vi "Read All.vi"(8 "error in (no error)":errorcluster, 11 "Flip Mirror Containter in":refnum<class "Flip Mirror Containter.lvclass">) -> (0 "error out":errorcluster, 2 "Mirrors-NP":T1, 3 "Flip Mirror Containter out":refnum<class "Flip Mirror Containter.lvclass">)   [LabVIEW 2016, in "Flip Mirror Containter.lvclass"]
uses:
  Flip Mirror Containter.lvclass
  Controls/Flip Mirrors.ctl
  Controls/Mirror Data.ctl
  Flip Mirror Containter.lvclass/Flip Mirror Containter.ctl
  SolarMir.lvclass
  ExtFlatMir.lvclass
  ThArMir.lvclass
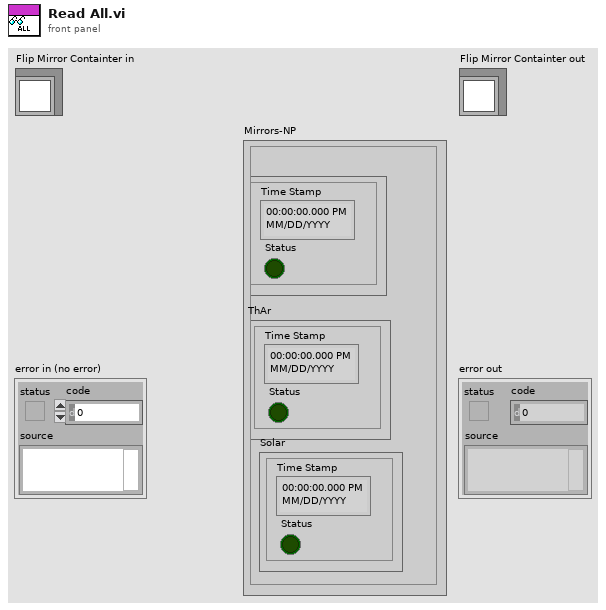
[diagram p1: front panel]
types:
  T1 = typedef "Flip Mirrors.ctl" = cluster{"ExtFlat":T2, "ThAr":T2, "Solar":T2}
  T2 = typedef "Mirror Data.ctl" = cluster{"Status":bool, "Time Stamp":timestamp}
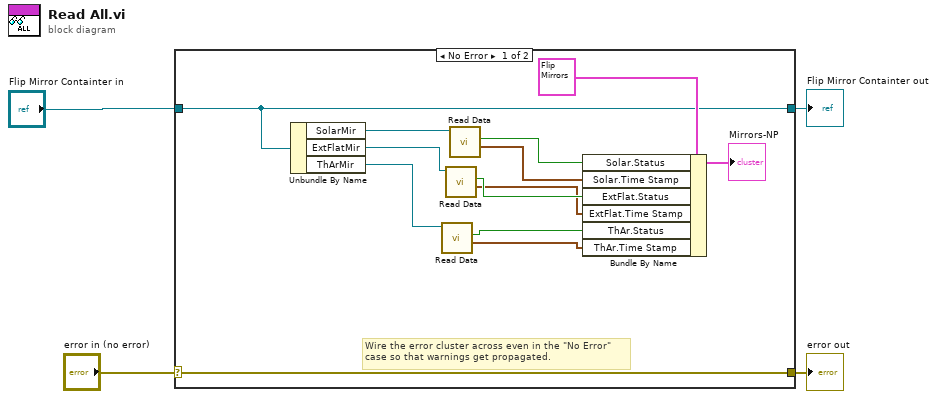
[diagram p0: block diagram]
diagram:
  n1 = case shown="No Error" "error in (no error)" {
    selector: "error in (no error)" -> [w17 w19]
    tunnel: [w17 w19] -> w3
    tunnel: [w12 w18] -> w1
    tunnel: "Flip Mirror Containter in" -> [w12 w18]
    frame No Error {
      # "Wire the error cluster across even in the \"No Error\"\ncase so that warnings get propagated."
      n2 = Unbundle By Name(w12) -> ("SolarMir"=w13:refnum<class "SolarMir.lvclass">, "ExtFlatMir"=w10:refnum<class "ExtFlatMir.lvclass">, "ThArMir"=w5:refnum<class "ThArMir.lvclass">)
      n3 = call-dynamic "Read Data.vi"("FlipMir in"=w5) -> ("Time Stamp"=w7:timestamp, "Status"=w6:bool)  [unwired: 7 in, 2 out]
      n4 = call-dynamic "Read Data.vi"("FlipMir in"=w10) -> ("Time Stamp"=w8:timestamp, "Status"=w9:bool)  [unwired: 7 in, 2 out]
      n5 = call-dynamic "Read Data.vi"("FlipMir in"=w13) -> ("Time Stamp"=w11:timestamp, "Status"=w14:bool)  [unwired: 7 in, 2 out]
      n6 = Bundle By Name(cluster=T1 {"ExtFlat"={"Status"=FALSE, "Time Stamp"=timestamp(0 s since 1904-01-01)}, "ThAr"={"Status"=FALSE, "Time Stamp"=timestamp(0 s since 1904-01-01)}, "Solar"={"Status"=FALSE, "Time Stamp"=timestamp(0 s since 1904-01-01)}} ("Mirrors"), "Solar.Status"=w14, "Solar.Time Stamp"=w11, "ExtFlat.Status"=w9, "ExtFlat.Time Stamp"=w8, "ThAr.Status"=w6, "ThAr.Time Stamp"=w7) -> (→"Mirrors-NP":T1)
    }
    frame Error {
    }
  }
  "error out" <- w3
  "Flip Mirror Containter out" <- w1
